vi "ToTable.vi"(8 "error in (no error)":errorcluster, 10 "variant":variant, 11 "node in":refnum<class "tag bus configurable plugin editor node.lvclass">) -> (0 "error out":errorcluster, 2 "table":string[][](array[string]), 3 "node in out":refnum<class "tag bus configurable plugin editor node.lvclass">)   [LabVIEW 2013, in "tag bus configurable plugin editor node.lvclass"]
doc: "Copyright 2015 National Instruments Corporation\n\nLicensed under the Apache License, Version 2.0 (the \"License\"); you may not use this file except in compliance with the License. You may obtain a copy of the License at http://www.apache.org/licenses/LICENSE-2.0\nUnless required by applicable law or agreed to in writing, software distributed under the License is distributed on an \"AS IS\" BASIS, WITHOUT WARRANTIES OR CONDITIONS OF ANY KIND, either express or implied. See the License for the specific language governing permissions and limitations under the License."
uses:
  tag bus configurable plugin editor node.lvclass
  <vilib>/NI/Module Execution Interface/Engine Configuration/engine configuration.lvclass
  tag bus configurable plugin editor node.lvclass/tag bus configurable plugin editor node.ctl
  module/configuration/tag bus configurable plugin module configuration.lvclass
  <vilib>/NI/Configuration Framework/serializable configuration/NISE_CEF_serializable configuration.lvclass/NISE_CEF_serializable configuration.ctl
  <vilib>/NI/Tag Bus Module Framework/channel/TBM channel.lvclass/TBM channel.ctl
  <vilib>/NI/Tag Bus/tag/tag descriptor.lvclass/tag descriptor.ctl
  <vilib>/Utility/LVClass/Get LV Class Name.vi
  <vilib>/NI/Configuration Framework/error generator/NISE_error generator.vi
  <vilib>/NI/Tag Bus/tag/tag descriptor.lvclass
  <vilib>/NI/Tag Bus Module Framework/channel/TBM channel.lvclass
  <vilib>/NI/Configuration Framework/serializable configuration/NISE_CEF_serializable configuration.lvclass
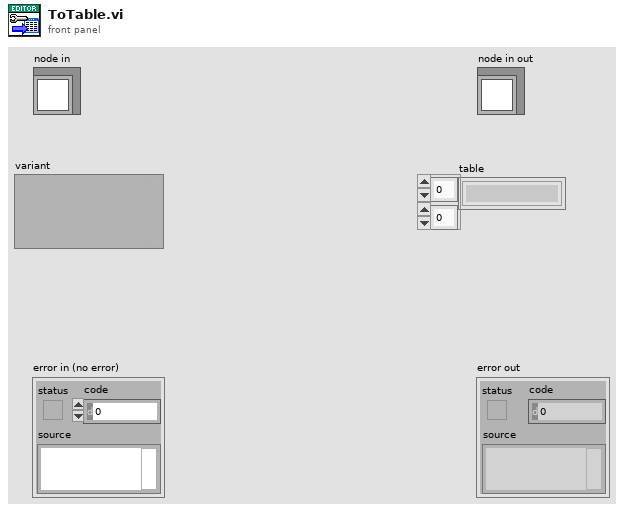
[diagram p1: front panel]
types:
  T1 = typedef "TBM channel.lvclass/channel classification.ctl" = enum16{"input data", "output data", "processing parameter", "processing result"}
  T2 = typedef "tag bus.lvlib/tag descriptor.lvclass/Data Type.ctl" = enum16{"Double", "Single", "I64", "I32", "I16", "I8", "U64", "U32", "U16", "U8", "Boolean", "String", "Array of Double", "Array of Single", "Array of I64", "Array of I32", "Array of I16", "Array of I8", "Array of U64", "Array of U32", "Array of U16", "Array of U8", "Array of Boolean", "Array of String"}
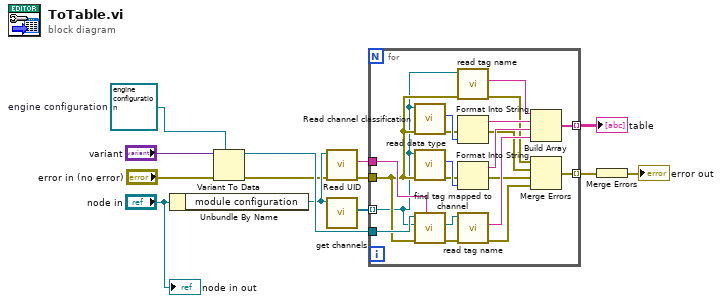
[diagram p0: block diagram]
diagram:
  w13 = refnum<class "engine configuration.lvclass"> refnum  # engine configuration
  n1 = Unbundle By Name("node in") -> ("module configuration"=w6:refnum<class "tag bus configurable plugin module configuration.lvclass">)
  n2 = Variant To Data(error in="error in (no error)", type=w13, Variant="variant") -> (data=w8:refnum<class "engine configuration.lvclass">, error out=w4:errorcluster)
  n3 = call <vilib>:"Read UID.vi"("error in"=w4, "configuration in"=w6) -> ("error out"=w3:errorcluster, "instance id"=w5:string)  [unwired: 7 in, 1 out]
  n4 = call-dynamic "get channels.vi"("module configuration in"=w6) -> ("channels"=w9:refnum<class "TBM channel.lvclass">[])  [unwired: 9 in, 1 out]
  n5 = for {
    tunnel: [w33] -> w10 mode=indexing
    tunnel: w9 -> [w14] mode=indexing
    tunnel: w8 -> [w30]
    tunnel: w5 -> [w24]
    tunnel: w3 -> [w23]
    tunnel: [w15] -> w2 mode=indexing
    n6 = call <vilib>:"Read channel classification.vi"("error in"=w23, "channel in"=w14) -> ("error out"=w21:errorcluster, "channel classification"=w29:T1)  [unwired: 7 in, 1 out]
    n7 = call <vilib>:"read data type.vi"("error in"=w23, "system tag in"=w14) -> ("error out"=w20:errorcluster, "data type"=w27:T2)  [unwired: 7 in, 1 out]
    n8 = call <vilib>:"find tag mapped to channel.vi"("owner"=w24, "error in"=w23, "channel"=w14, "engine configuration in"=w30) -> ("error out"=w22:errorcluster, "tag"=w32:refnum<class "tag descriptor.lvclass">)  [unwired: 5 in, 1 out]
    n9 = call <vilib>:"read tag name.vi"("error in"=w23, "system tag in"=w14) -> ("error out"=w16:errorcluster, "name"=w25:string)  [unwired: 7 in, 1 out]
    n10 = Format Into String(error in=w21, w29) -> (resulting string=w28:string, error out=w17:errorcluster)  [unwired: 2 in]
    n11 = Format Into String(error in=w20, w27) -> (resulting string=w26:string, error out=w18:errorcluster)  [unwired: 2 in]
    n12 = call <vilib>:"read tag name.vi"("error in"=w22, "system tag in"=w32) -> ("error out"=w19:errorcluster, "name"=w31:string)  [unwired: 7 in, 1 out]
    n13 = Build Array(w25, w28, w26, w31) -> (w33:string[])
    n14 = Merge Errors(w16, w17, w18, w19) -> (w15:errorcluster)
  }
  "table" <- w10
  n15 = Merge Errors(w2) -> (→"error out":errorcluster)
  "node in out" <- "node in"
